vi "Sigma_Delta_Simulation.vi"() -> ()   [LabVIEW 2016]
uses:
  <vilib>/Analysis/2dsp.llb/Real FFT.vi
  <vilib>/Analysis/NI_AALPro.lvlib
panel:
  out "subarray":dbl[](array[numeric])
  out "Waveform Graph 2":dbl[](graph)=[-1.0, 260.05238444010314, 516.6380902050414, 764.3668647301795, 998.9999999999998, 1216.5228580174412, 1413.2135623730946, 1585.7066805824702, 1731.0508075688767, 1846.7590650225734, 1930.851652578136, 1981.8897227476207, 1998.9999999999995, 1981.889722747621, 1930.8516525781363, 1846.7590650225739, 1731.0508075688772, 1585.7066805824709, 1413.213562373095, 1216.522858017442, 999.0000000000003, 764.3668647301804, 516.6380902050421, 260.05238444010405, -0.9999999999992042, -262.05238444010234, -518.6380902050406, -766.3668647301788, -1000.999999999999, -1218.5228580174407, -1415.2135623730942, -1587.70668058247, -1733.0508075688765, -1848.7590650225734, -1932.851652578136, -1983.889722747621, -2000.9999999999998, -1983.8897227476211, -1932.8516525781367, -1848.759065022574, -1733.0508075688779, -1587.706680582471, -1415.213562373096, -1218.5228580174423, -1001.0000000000013, -766.3668647301809, -518.638090205043, -262.0523844401046, -1.0, 260.05238444010314, 516.6380902050414, 764.3668647301795, 998.9999999999998, 1216.5228580174412, 1413.2135623730946, 1585.7066805824702, 1731.0508075688767, 1846.7590650225734, 1930.851652578136, 1981.8897227476207, 1998.9999999999995, 1981.889722747621, 1930.8516525781363, 1846.7590650225739, 1731.0508075688772, 1585.7066805824709, 1413.213562373095, 1216.522858017442, 999.0000000000003, 764.3668647301804, 516.6380902050421, 260.05238444010405, -0.9999999999992042, -262.05238444010234, -518.6380902050406, -766.3668647301788, -1000.999999999999, -1218.5228580174407, -1415.2135623730942, -1587.70668058247, -1733.0508075688765, -1848.7590650225734, -1932.851652578136, -1983.889722747621, -2000.9999999999998, -1983.8897227476211, -1932.8516525781367, -1848.759065022574, -1733.0508075688779, -1587.706680582471, -1415.213562373096, -1218.5228580174423, -1001.0000000000013, -766.3668647301809, -518.638090205043, -262.0523844401046, -1.0, 260.05238444010314, 516.6380902050414, 764.3668647301795, 998.9999999999998, 1216.5228580174412, 1413.2135623730946, 1585.7066805824702, 1731.0508075688767, 1846.7590650225734, 1930.851652578136, 1981.8897227476207, 1998.9999999999995, 1981.889722747621, 1930.8516525781363, 1846.7590650225739, 1731.0508075688772, 1585.7066805824709, 1413.213562373095, 1216.522858017442, 999.0000000000003, 764.3668647301804, 516.6380902050421, 260.05238444010405, -0.9999999999992042, -262.05238444010234, -518.6380902050406, -766.3668647301788, -1000.999999999999, -1218.5228580174407, -1415.2135623730942, -1587.70668058247, -1733.0508075688765, -1848.7590650225734, -1932.851652578136, -1983.889722747621, -2000.9999999999998, -1983.8897227476211, -1932.8516525781367, -1848.759065022574, -1733.0508075688779, -1587.706680582471, -1415.213562373096, -1218.5228580174423, -1001.0000000000013, -766.3668647301809, -518.638090205043, -262.0523844401046, -1.0, 260.05238444010314, 516.6380902050414, 764.3668647301795, 998.9999999999998, 1216.5228580174412, 1413.2135623730946, 1585.7066805824702, 1731.0508075688767, 1846.7590650225734, 1930.851652578136, 1981.8897227476207, 1998.9999999999995, 1981.889722747621, 1930.8516525781363, 1846.7590650225739, 1731.0508075688772, 1585.7066805824709, 1413.213562373095, 1216.522858017442, 999.0000000000003, 764.3668647301804, 516.6380902050421, 260.05238444010405, -0.9999999999992042, -262.05238444010234, -518.6380902050406, -766.3668647301788, -1000.999999999999, -1218.5228580174407, -1415.2135623730942, -1587.70668058247, -1733.0508075688765, -1848.7590650225734, -1932.851652578136, -1983.889722747621, -2000.9999999999998, -1983.8897227476211, -1932.8516525781367, -1848.759065022574, -1733.0508075688779, -1587.706680582471, -1415.213562373096, -1218.5228580174423, -1001.0000000000013, -766.3668647301809, -518.638090205043, -262.0523844401046, -1.0, 260.05238444010314, 516.6380902050414, 764.3668647301795, 998.9999999999998, 1216.5228580174412, 1413.2135623730946, 1585.7066805824702, 1731.0508075688767, 1846.7590650225734, 1930.851652578136, 1981.8897227476207, 1998.9999999999995, 1981.889722747621, 1930.8516525781363, 1846.7590650225739, 1731.0508075688772, 1585.7066805824709, 1413.213562373095, 1216.522858017442, 999.0000000000003, 764.3668647301804, 516.6380902050421, 260.05238444010405, -0.9999999999992042, -262.05238444010234, -518.6380902050406, -766.3668647301788, -1000.999999999999, -1218.5228580174407, -1415.2135623730942, -1587.70668058247, -1733.0508075688765, -1848.7590650225734, -1932.851652578136, -1983.889722747621, -2000.9999999999998, -1983.8897227476211, -1932.8516525781367, -1848.759065022574, -1733.0508075688779, -1587.706680582471, -1415.213562373096, -1218.5228580174423, -1001.0000000000013, -766.3668647301809, -518.638090205043, -262.0523844401046, -1.0, 260.05238444010314, 516.6380902050414, 764.3668647301795, 998.9999999999998, 1216.5228580174412, 1413.2135623730946, 1585.7066805824702, 1731.0508075688767, 1846.7590650225734, 1930.851652578136, 1981.8897227476207, 1998.9999999999995, 1981.889722747621, 1930.8516525781363, 1846.7590650225739, 1731.0508075688772, 1585.7066805824709, 1413.213562373095, 1216.522858017442, 999.0000000000003, 764.3668647301804, 516.6380902050421, 260.05238444010405, -0.9999999999992042, -262.05238444010234, -518.6380902050406, -766.3668647301788, -1000.999999999999, -1218.5228580174407, -1415.2135623730942, -1587.70668058247, -1733.0508075688765, -1848.7590650225734, -1932.851652578136, -1983.889722747621, -2000.9999999999998, -1983.8897227476211, -1932.8516525781367, -1848.759065022574, -1733.0508075688779, -1587.706680582471, -1415.213562373096, -1218.5228580174423, -1001.0000000000013, -766.3668647301809, -518.638090205043, -262.0523844401046, -1.0, 260.05238444010314, 516.6380902050414, 764.3668647301795, 998.9999999999998, 1216.5228580174412, 1413.2135623730946, 1585.7066805824702, 1731.0508075688767, 1846.7590650225734, 1930.851652578136, 1981.8897227476207, 1998.9999999999995, 1981.889722747621, 1930.8516525781363, 1846.7590650225739, 1731.0508075688772, 1585.7066805824709, 1413.213562373095, 1216.522858017442, 999.0000000000003, 764.3668647301804, 516.6380902050421, 260.05238444010405, -0.9999999999992042, -262.05238444010234, -518.6380902050406, -766.3668647301788, -1000.999999999999, -1218.5228580174407, -1415.2135623730942, -1587.70668058247, -1733.0508075688765, -1848.7590650225734, -1932.851652578136, -1983.889722747621, -2000.9999999999998, -1983.8897227476211, -1932.8516525781367, -1848.759065022574, -1733.0508075688779, -1587.706680582471, -1415.213562373096, -1218.5228580174423, -1001.0000000000013, -766.3668647301809, -518.638090205043, -262.0523844401046, -1.0, 260.05238444010314, 516.6380902050414, 764.3668647301795, 998.9999999999998, 1216.5228580174412, 1413.2135623730946, 1585.7066805824702, 1731.0508075688767, 1846.7590650225734, 1930.851652578136, 1981.8897227476207, 1998.9999999999995, 1981.889722747621, 1930.8516525781363, 1846.7590650225739, 1731.0508075688772, 1585.7066805824709, 1413.213562373095, 1216.522858017442, 999.0000000000003, 764.3668647301804, 516.6380902050421, 260.05238444010405, -0.9999999999992042, -262.05238444010234, -518.6380902050406, -766.3668647301788, -1000.999999999999, -1218.5228580174407, -1415.2135623730942, -1587.70668058247, -1733.0508075688765, -1848.7590650225734, -1932.851652578136, -1983.889722747621, -2000.9999999999998, -1983.8897227476211, -1932.8516525781367, -1848.759065022574, -1733.0508075688779, -1587.706680582471, -1415.213562373096, -1218.5228580174423, -1001.0000000000013, -766.3668647301809, -518.638090205043, -262.0523844401046, -1.0, 260.05238444010314, 516.6380902050414, 764.3668647301795, 998.9999999999998, 1216.5228580174412, 1413.2135623730946, 1585.7066805824702, 1731.0508075688767, 1846.7590650225734, 1930.851652578136, 1981.8897227476207, 1998.9999999999995, 1981.889722747621, 1930.8516525781363, 1846.7590650225739, 1731.0508075688772, 1585.7066805824709, 1413.213562373095, 1216.522858017442, 999.0000000000003, 764.3668647301804, 516.6380902050421, 260.05238444010405, -0.9999999999992042, -262.05238444010234, -518.6380902050406, -766.3668647301788, -1000.999999999999, -1218.5228580174407, -1415.2135623730942, -1587.70668058247, -1733.0508075688765, -1848.7590650225734, -1932.851652578136, -1983.889722747621, -2000.9999999999998, -1983.8897227476211, -1932.8516525781367, -1848.759065022574, -1733.0508075688779, -1587.706680582471, -1415.213562373096, -1218.5228580174423, -1001.0000000000013, -766.3668647301809, -518.638090205043, -262.0523844401046, -1.0, 260.05238444010314, 516.6380902050414, 764.3668647301795, 998.9999999999998, 1216.5228580174412, 1413.2135623730946, 1585.7066805824702, 1731.0508075688767, 1846.7590650225734, 1930.851652578136, 1981.8897227476207, 1998.9999999999995, 1981.889722747621, 1930.8516525781363, 1846.7590650225739, 1731.0508075688772, 1585.7066805824709, 1413.213562373095, 1216.522858017442, 999.0000000000003, 764.3668647301804, 516.6380902050421, 260.05238444010405, -0.9999999999992042, -262.05238444010234, -518.6380902050406, -766.3668647301788, -1000.999999999999, -1218.5228580174407, -1415.2135623730942, -1587.70668058247, -1733.0508075688765, -1848.7590650225734, -1932.851652578136, -1983.889722747621, -2000.9999999999998, -1983.8897227476211, -1932.8516525781367, -1848.759065022574, -1733.0508075688779, -1587.706680582471, -1415.213562373096, -1218.5228580174423, -1001.0000000000013, -766.3668647301809, -518.638090205043, -262.0523844401046]
  in  "C1":dbl=1.0
  in  "C2":dbl
  in  "C3":dbl
  in  "B1":dbl=2047.0
  in  "B2":dbl
  in  "B3":dbl
  in  "X Axes Log":bool
  in  "Tab Control":enum32{"Zeitberich", "Output", "FFT"}(tab)=enum."Output"
  out "Waveform Graph":dbl[][](graph)
  out "Waveform Graph 3":dbl[](graph)
  out "XY Graph":cluster{dbl[], dbl[]}(graph)
  in  "AutoPlay":bool
  in  "Play":bool
  in  "OutputTime":u8=2
  out "error out":errorcluster
  in  "stop":bool
  in  "A3":dbl
  in  "#samples":i32=48
  in  "FSsine_in":i32=48000
  out "Fsine_in":dbl=1000.0
  in  "Feedback":dbl=2047.0
  in  "A1":dbl=3070.0
  in  "A2":dbl
  in  "Cycles":i32=10
  in  "amplitude":u32=2000 format="%x"
  in  "Oversampling":i32=31
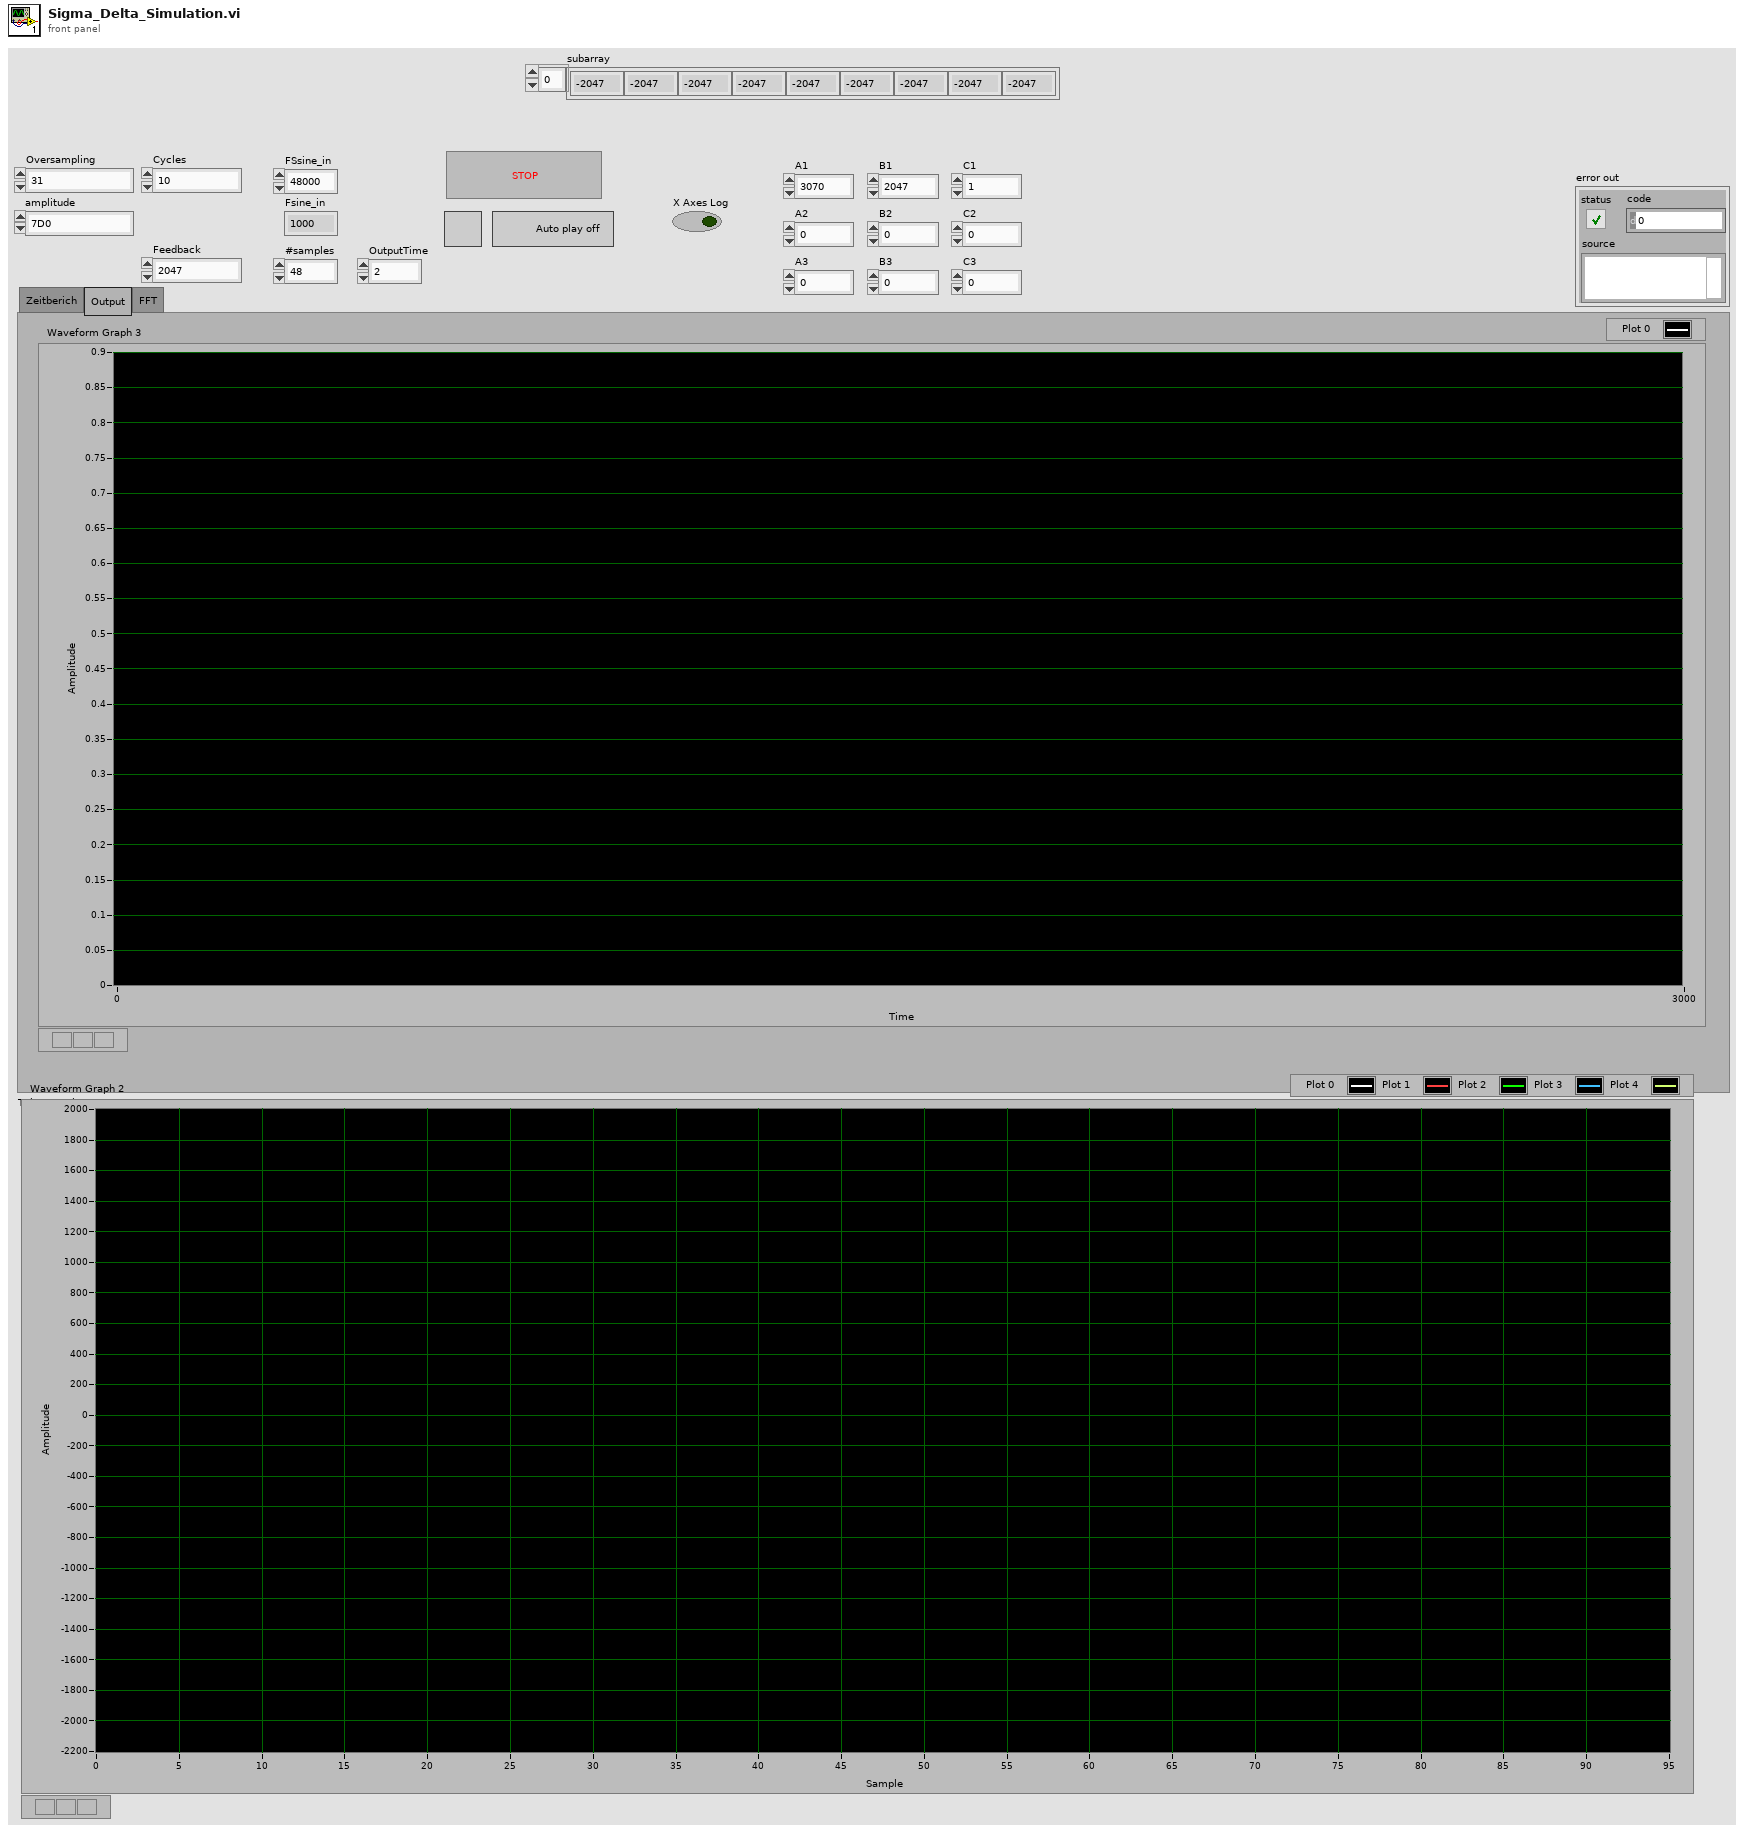
[diagram p1: front panel]
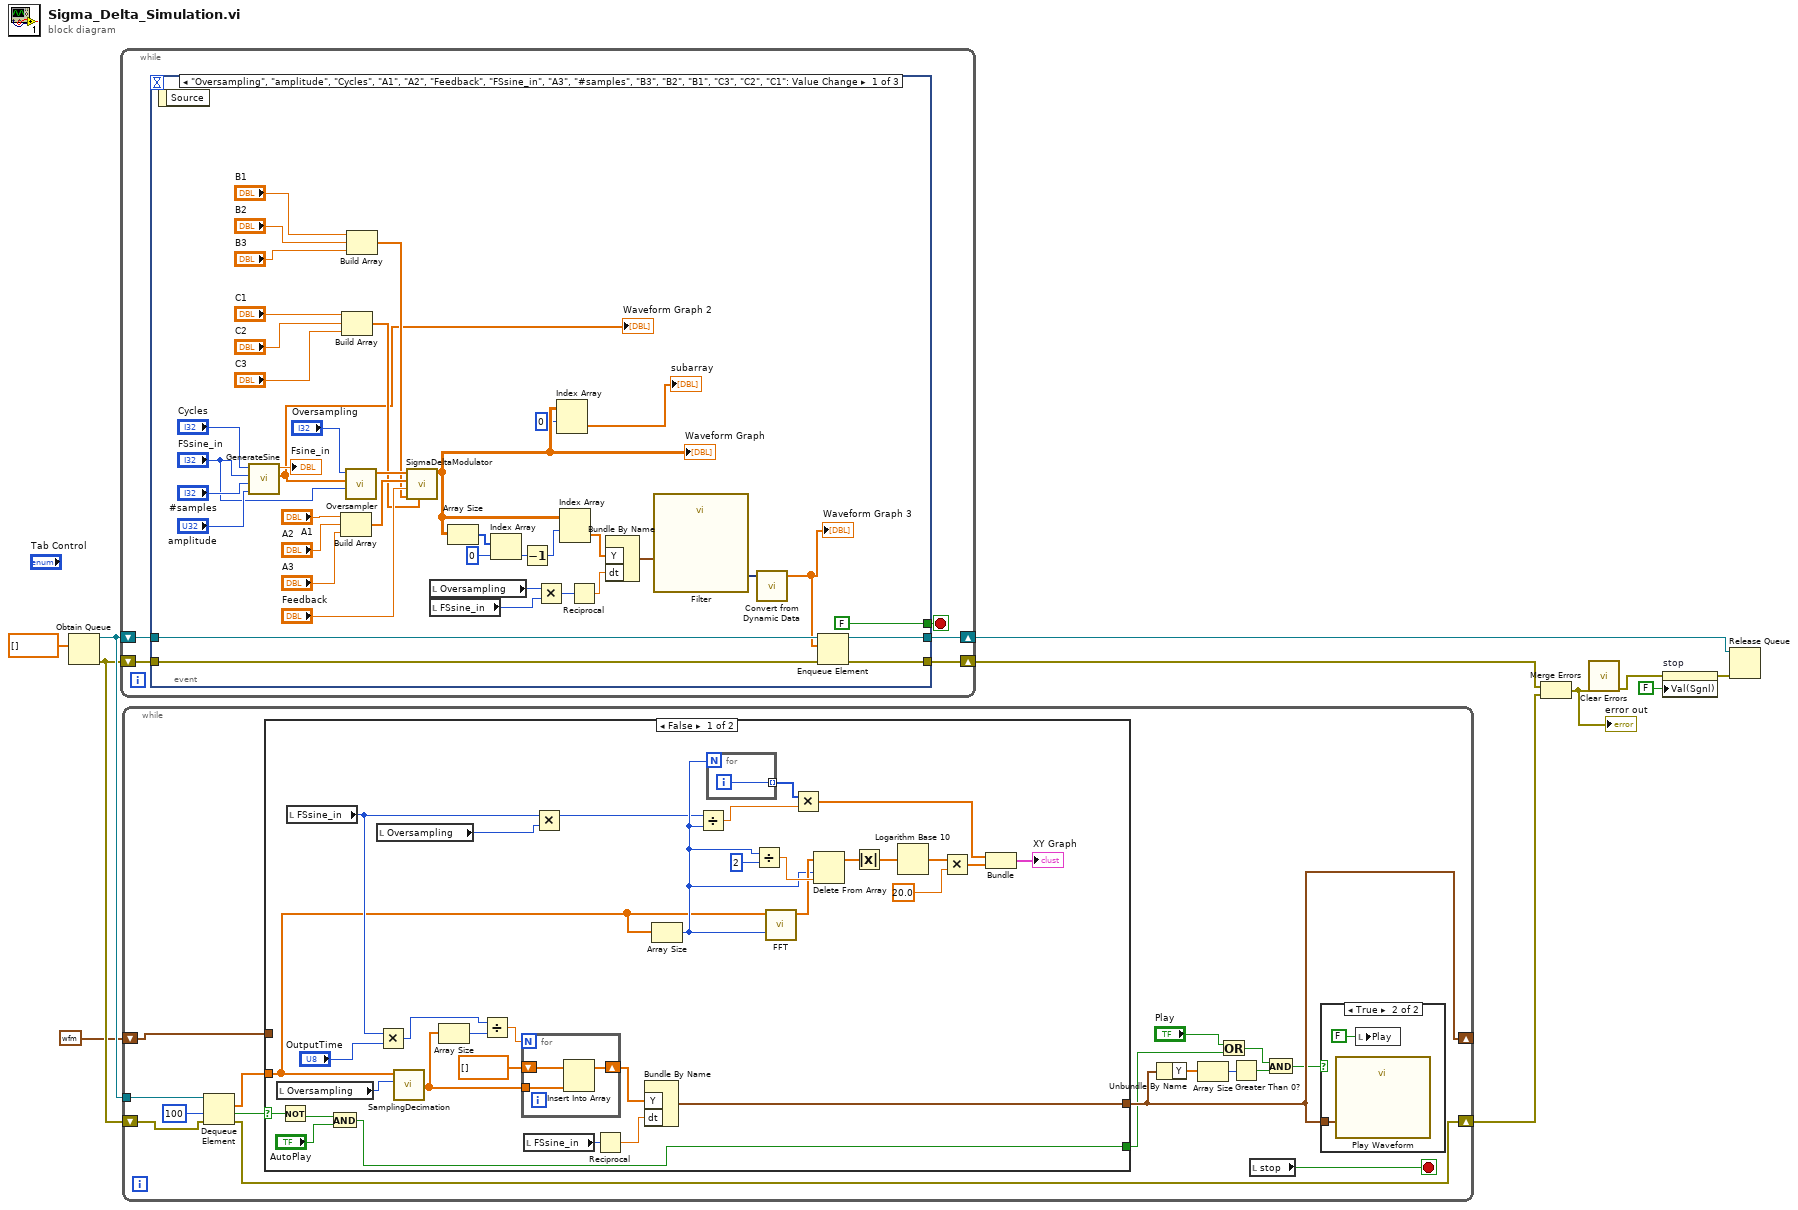
[diagram p0: block diagram]
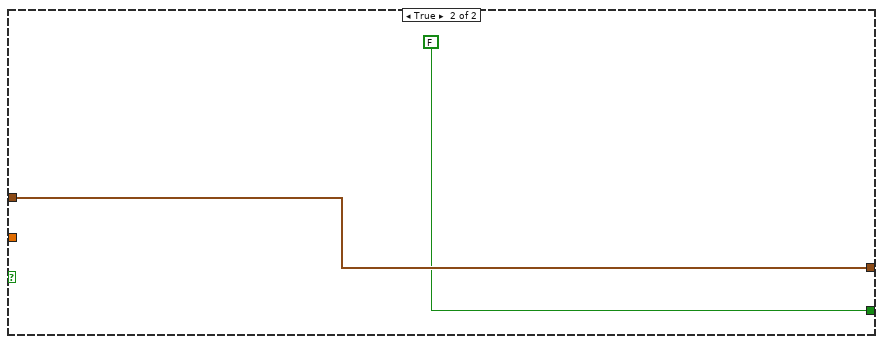
[diagram p2: hidden frame]
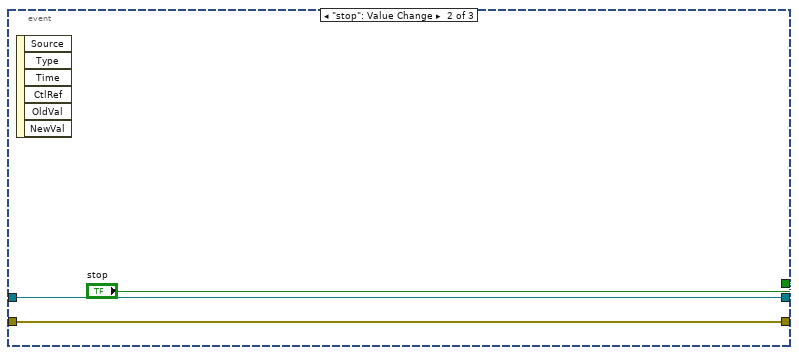
[diagram p4: hidden frame]
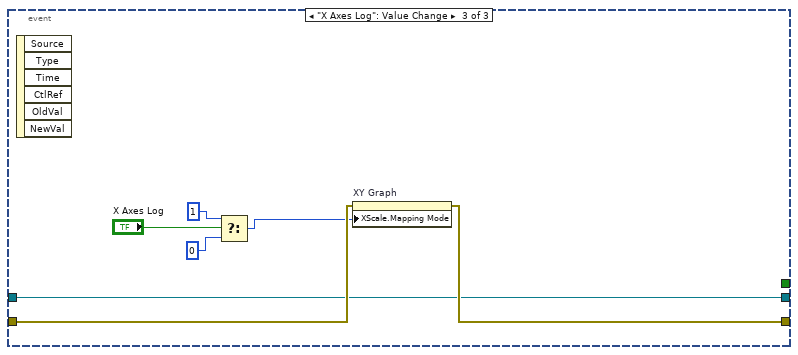
[diagram p5: hidden frame]
diagram:
  n1 = Obtain Queue(element data type=dbl[] []) -> (queue out=w10:refnum<queue>, error out=w9:errorcluster)  [unwired: 4 in, 1 out]
  n2 = while {
    shift-right: [w14] -> w8
    shift-left: w9 -> [w13]
    shift-right: [w12] -> w2
    shift-left: w10 -> [w15]
    stop <- w16 stop-if-true
    n3 = event shown="[0] \"Oversampling\", \"amplitude\", \"Cycles\", \"A1\", \"A2\", \"Feedback\", \"FSsine_in\", \"A3\", \"#samples\", \"B3\", \"B2\", \"B1\", \"C3\", \"C2\", \"C1\": Value Change" {
      selector: _ -> [_ _ _]
      dyn-events: _ -> [_ _ _]
      timeout: _ -> [_ _ _]
      tunnel: [FALSE "stop" _] -> w16
      tunnel: w13 -> [w54 w59 w67]
      tunnel: w15 -> [w56 w58 w65]
      tunnel: [w55 w59 w66] -> w14
      tunnel: [w53 w58 w65] -> w12
      event "Oversampling", "amplitude", "Cycles", "A1", "A2", "Feedback", "FSsine_in", "A3", "#samples", "B3", "B2", "B1", "C3", "C2", "C1": Value Change {
        n4 = event-data() -> ()  [unwired: 1 in, 1 out]
        n5 = call "GenerateSine.vi"("amplitude"="amplitude", "#samples"="#samples", "FSsine_in"="FSsine_in", "Cycles"="Cycles") -> ("Array"=w22:dbl[], "Fsine_in"=→"Fsine_in":dbl)  [unwired: 6 in]
        "Waveform Graph 2" <- w22
        n6 = Build Array("A1", "A2", "A3") -> (w44:dbl[])
        n7 = Build Array("C1", "C2", "C3") -> (w29:dbl[])
        n8 = call "Oversampler.vi"("Samplerate"="FSsine_in", "Array in"=w22, "Oversampling"="Oversampling") -> ("Array out"=w43:dbl[])  [unwired: 8 in]
        n9 = Build Array("B1", "B2", "B3") -> (w30:dbl[])
        n10 = call "SigmaDeltaModulator.vi"("Coef.c"=w29, "Coef.b"=w30, "FeedbackVal"="Feedback", "Coef.a"=w44, "InputData"=w43) -> ("OutputData"=w19:dbl[][])  [unwired: 6 in]
        "Waveform Graph" <- w19
        n11 = local read "Oversampling"() -> (w39:i32)
        n12 = local read "FSsine_in"() -> (w38:i32)
        n13 = Array Size(array=w19) -> (size(s)=w36:i32[])
        n14 = Index Array(array=w36, index=0) -> (element=w35:i32)
        n15 = Decrement(x=w35) -> (x-1=w33:i32)
        n16 = Multiply(x=w39, y=w38) -> (x*y=w37:i32)
        n17 = Index Array(array=w19, index (row)=0) -> (element=→"subarray":dbl[])  [unwired: 1 in]
        n18 = Index Array(array=w19, index (row)=w33) -> (element=w21:dbl[])  [unwired: 1 in]
        n19 = Reciprocal(x=w37) -> (1/x=w41:dbl)
        n20 = Bundle By Name("Y"=w21, "dt"=w41) -> (w42:waveform(dbl))  [unwired: 1 in]
        n21 = call "Filter"("Signal"=w42) -> ("Filtered Signal"=w40:dynamicdata)  [unwired: 9 in, 1 out]
        n22 = call "Convert from Dynamic Data"("Dynamic Data Type"=w40) -> ("Array"=w20:dbl[])  [unwired: 3 in]
        "Waveform Graph 3" <- w20
        n23 = Enqueue Element(queue=w56, element=w20, error in (no error)=w54) -> (queue out=w53:refnum<queue>, error out=w55:errorcluster)  [unwired: 1 in, 1 out]
      }
      event "stop": Value Change {
        n24 = event-data() -> ()  [unwired: 1 in, 6 out]
      }
      event "X Axes Log": Value Change {
        n25 = event-data() -> ()  [unwired: 1 in, 6 out]
        n26 = Select(t=u8 1, s="X Axes Log", f=u8 0) -> (s? t:f=w63:u8)
        n27 = property on="XY Graph" class="XYGraph (strict)"(error in=w67, "XScale.Mapping Mode"=w63) -> (error out=w66:errorcluster)  [unwired: 1 in, 1 out]
      }
    }
  }
  n28 = while {
    tunnel: w10 -> [w83]
    shift-right: [w81] -> w7
    shift-left: w9 -> [w82]
    shift-right: [w75] -> _
    shift-left: waveform(dbl) {"t0"=timestamp(0 s since 1904-01-01), "dt"=1.0, "Y"=[]} -> [w76]
    stop <- w80 stop-if-true
    n29 = Dequeue Element(queue=w83, timeout in ms (-1)=100, error in (no error)=w82) -> (element=w77:dbl[], timed out?=w79:bool, error out=w81:errorcluster)  [unwired: 1 out]
    n30 = case shown="False" w79 {
      selector: w79 -> [w105 _]
      tunnel: w77 -> [w84 _]
      tunnel: [w108 w121] -> w75
      tunnel: w76 -> [_ w121]
      tunnel: [w103 FALSE] -> w68
      frame False {
        n31 = local read "Oversampling"() -> (w114:i32)
        n32 = Not(x=w105) -> (.not. x?=w102:bool)
        n33 = local read "FSsine_in"() -> (w94:i32)
        n34 = And(x=w102, y="AutoPlay") -> (x .and. y?=w103:bool)
        n35 = local read "Oversampling"() -> (w85:i32)
        n36 = Multiply(x=w94, y="OutputTime") -> (x*y=w110:i32)
        n37 = call "SamplingDecimation.vi"("Dezimation"=w114, "InputData"=w84) -> ("OutputData"=w113:dbl[])  [unwired: 9 in]
        n38 = Array Size(array=w113) -> (size(s)=w111:i32)
        n39 = Divide(x=w110, y=w111) -> (x/y=w109:dbl)
        n40 = for {
          N: w109 -> [_]
          shift-right: [w118] -> w87
          shift-left: dbl[] [] -> [w119]
          tunnel: w113 -> [w117]
          n41 = Insert Into Array(array=w119, new element=w117) -> (w118:dbl[])  [unwired: 1 in]
        }
        n42 = local read "FSsine_in"() -> (w107:i32)
        n43 = Multiply(x=w94, y=w85) -> (x*y=w86:i32)
        n44 = Reciprocal(x=w107) -> (1/x=w106:dbl)
        n45 = Bundle By Name("Y"=w87, "dt"=w106) -> (w108:waveform(dbl))  [unwired: 1 in]
        n46 = Array Size(array=w84) -> (size(s)=w93:i32)
        n47 = Divide(x=w86, y=w93) -> (x/y=w91:dbl)
        n48 = for {
          N: w93 -> [_]
          tunnel: [w116] -> w92 mode=indexing
          i -> [w116]
        }
        n49 = Divide(x=w93, y=2) -> (x/y=w97:dbl)
        n50 = call-poly <vilib>:"FFT.vi"("FFT size"=w93, "X"=w84) -> ("FFT {X}"=w96:cdb[])  [unwired: 8 in, 1 out]
        n51 = Multiply(x=w92, y=w91) -> (x*y=w90:dbl[])
        n52 = Delete From Array(array=w96, length=w93, index=w97) -> (array with subset deleted=w95:cdb[])  [unwired: 1 out]
        n53 = Absolute Value(x=w95) -> (abs(x)=w101:dbl[])
        n54 = Logarithm Base 10(1:w101) -> (0:w100:dbl[])
        n55 = Multiply(x=w100, y=20.0) -> (x*y=w89:dbl[])
        n56 = Bundle(w90, w89) -> (→"XY Graph":cluster{dbl[], dbl[]})  [unwired: 1 in]
      }
      frame True {
      }
    }
    n57 = Unbundle By Name(w75) -> ("Y"=w73:dbl[])
    n58 = Array Size(array=w73) -> (size(s)=w74:i32)
    n59 = Or(x="Play", y=w68) -> (x .or. y?=w69:bool)
    n60 = Greater Than 0?(x=w74) -> (x > 0?=w71:bool)
    n61 = local read "stop"() -> (w80:bool)
    n62 = And(x=w69, y=w71) -> (x .and. y?=w72:bool)
    n63 = case shown="True" w72 {
      tunnel: w75 -> [_ w123]
      frame False {
      }
      frame True {
        n64 = call "Play Waveform"("Data"=w123) -> ()  [unwired: 18 in, 1 out]
        n65 = local write "Play"(FALSE ("Play")) -> ()
      }
    }
  }
  n66 = Merge Errors(w8, w7) -> (w6:errorcluster)
  "error out" <- w6
  n67 = call <vilib>:"Clear Errors.vi"("error in (no error)"=w6) -> ("error out"=w4:errorcluster)  [unwired: 5 in, 1 out]
  n68 = property on="stop" class="Bool (strict)"(error in=w4, "Val(Sgnl)"=FALSE ("Value (Signaling)")) -> (error out=w3:errorcluster)  [unwired: 1 in, 1 out]
  n69 = Release Queue(queue=w2, error in (no error)=w3) -> ()  [unwired: 1 in, 3 out]
